vi "calc_coag_dose.vi"(10 "Enum":T1=enum."Target", 11 "RowData input":T2) -> (5 "RowData output":T2)   [LabVIEW 2019]
uses:
  RowData_Type.ctl
  enum_observed_clarified.ctl
  give_data_NR.ctl
  <vilib>/gmath/zero.llb/Newton Raphson Zero Finder (VI).vi
  <vilib>/gmath/NI_Gmath.lvlib
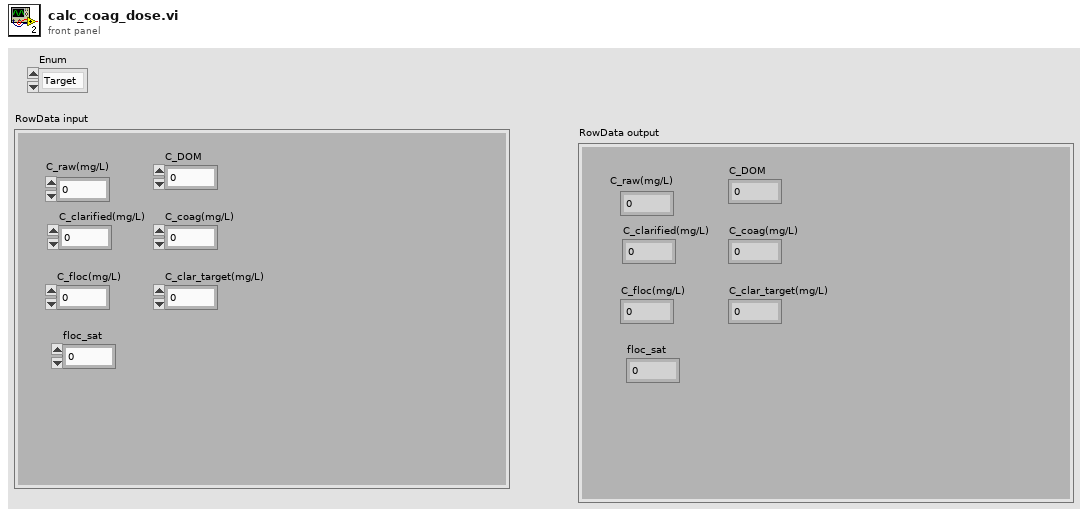
[diagram p1: front panel]
types:
  T1 = typedef "enum_observed_clarified.ctl" = enum16{"Observed", "Target"}
  T2 = typedef "RowData_Type.ctl" = cluster{"C_raw(mg/L)":dbl, "C_clarified(mg/L)":dbl, "C_floc(mg/L)":dbl, "floc_sat":dbl, "C_DOM":dbl, "C_coag(mg/L)":dbl, "C_clar_target(mg/L)":dbl}
  T3 = typedef "give_data_NR.ctl" = cluster{"RowData":T2, "Enum":T1}
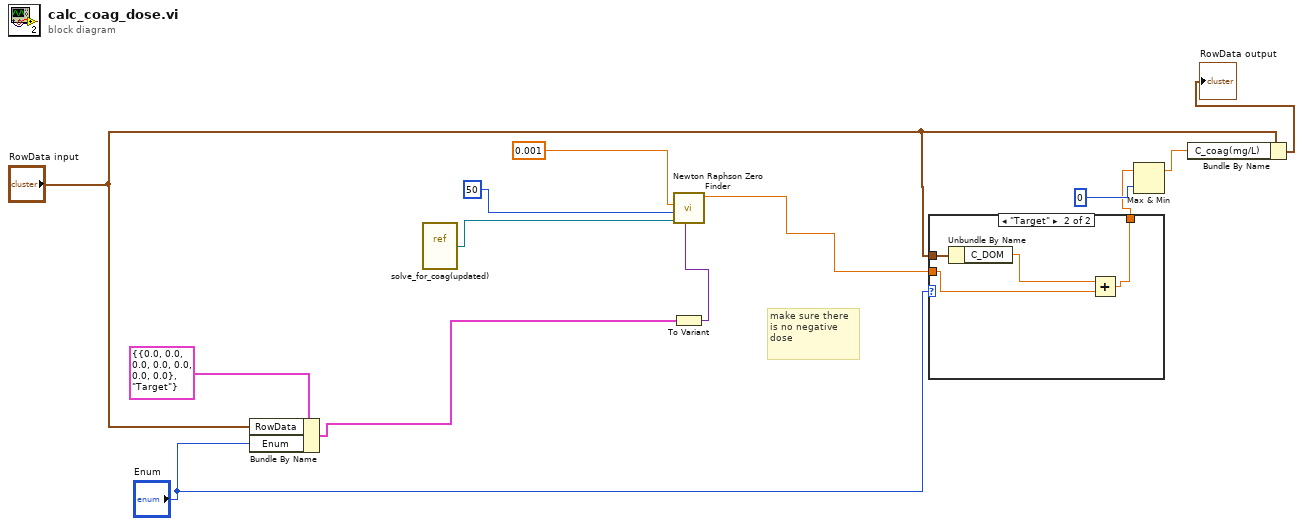
[diagram p0: block diagram]
diagram:
  # "make sure there is no negative dose"
  n1 = Bundle By Name(cluster=T3 {"RowData"={"C_raw(mg/L)"=0.0, "C_clarified(mg/L)"=0.0, "C_floc(mg/L)"=0.0, "floc_sat"=0.0, "C_DOM"=0.0, "C_coag(mg/L)"=0.0, "C_clar_target(mg/L)"=0.0}, "Enum"=enum."Target"} ("data to NR"), "RowData"="RowData input", "Enum"="Enum") -> (w7:T3)
  n2 = vi-ref "solve_for_coag(updated).vi"() -> (w10:refnum<vi>)
  n3 = To Variant(anything=w7) -> (Variant=w9:variant)
  n4 = call-poly <vilib>:"Newton Raphson Zero Finder.vi"("data"=w9, "f(x)"=w10, "end"=50, "start"=0.001) -> ("zero"=w5:dbl)  [unwired: 4 in, 3 out]
  n5 = case shown="\"Target\"" "Enum" {
    tunnel: "RowData input" -> [_ w18]
    tunnel: [w14 w16] -> w3
    tunnel: w5 -> [w14 w15]
    frame "Observed", Default {
    }
    frame "Target" {
      n6 = Unbundle By Name(w18) -> ("C_DOM"=w17:dbl)
      n7 = Add(x=w17, y=w15) -> (x+y=w16:dbl)
    }
  }
  n8 = Max & Min(x=w3, y=0) -> (max(x,y)=w2:dbl)  [unwired: 1 out]
  n9 = Bundle By Name(cluster="RowData input", "C_coag(mg/L)"=w2) -> (→"RowData output":T2)
